vi "MGI Read Spreadsheet File.vi"(5 "Dialog pattern (*.txt)":string="*.txt", 6 "Start Offset":i64, 7 "Delimiter (Tab)":string="\t", 8 "Error In":errorcluster, 11 "Path":path) -> (0 "Error Out":errorcluster, 1 "EOF Reached?":bool, 2 "Values":dbl[][](array[numeric]) format="%_3p", 3 "Headers":string[][](array[string]), 4 "End Offset":i64)   [LabVIEW 2016]
doc: "Reads a spreadsheet file by returning the first non-empty, non numeric containing rows as a header, then the following numeric rows. Reading starts at Start Offset. End Offset is the file offset for the next Header/Values section.\nThis VI is similar to the vi.lib file \"Read From Spreadsheet File.vi\", but it supports headers.\n\nAuthored by Shawn Walpole\nsupport@mooregoodideas.com\nwww.mooregoodideas.com\n\nCopyright (c) 2010, Moore Good Ideas, Inc.\n\nAll rights reserved.\n\nRedistribution and use in source and binary forms, with or without modification, are permitted provided that the following conditions are met:\n\n * Redistributions of source code must retain the above copyright notice, this list of conditions and the following disclaimer.\n * Redistributions in binary form must reproduce the above copyright notice, this list of conditions and the following disclaimer in the documentation and/or other materials provided with the distribution.\n * Neither the name of Moore Good Ideas, Inc. nor the names of its contributors may be used to endorse or promote products derived from this software without specific prior written permission.\n\nTHIS SOFTWARE IS PROVIDED BY THE COPYRIGHT HOLDERS AND CONTRIBUTORS \"AS IS\" AND ANY EXPRESS OR IMPLIED WARRANTIES, INCLUDING, BUT NOT LIMITED TO, THE IMPLIED WARRANTIES OF MERCHANTABILITY AND FITNESS FOR A PARTICULAR PURPOSE ARE DISCLAIMED. IN NO EVENT SHALL THE COPYRIGHT OWNER OR CONTRIBUTORS BE LIABLE FOR ANY DIRECT, INDIRECT, INCIDENTAL, SPECIAL, EXEMPLARY, OR CONSEQUENTIAL DAMAGES (INCLUDING, BUT NOT LIMITED TO, PROCUREMENT OF SUBSTITUTE GOODS OR SERVICES; LOSS OF USE, DATA, OR PROFITS; OR BUSINESS INTERRUPTION) HOWEVER CAUSED AND ON ANY THEORY OF LIABILITY, WHETHER IN CONTRACT, STRICT LIABILITY, OR TORT (INCLUDING NEGLIGENCE OR OTHERWISE) ARISING IN ANY WAY OUT OF THE USE OF THIS SOFTWARE, EVEN IF ADVISED OF THE POSSIBILITY OF SUCH DAMAGE."
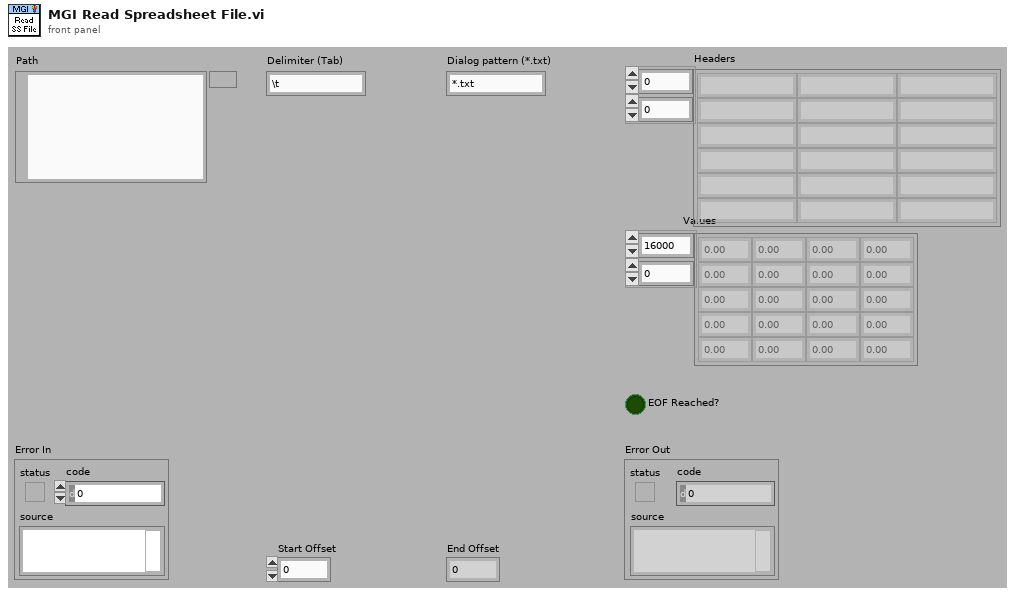
[diagram p1: front panel]
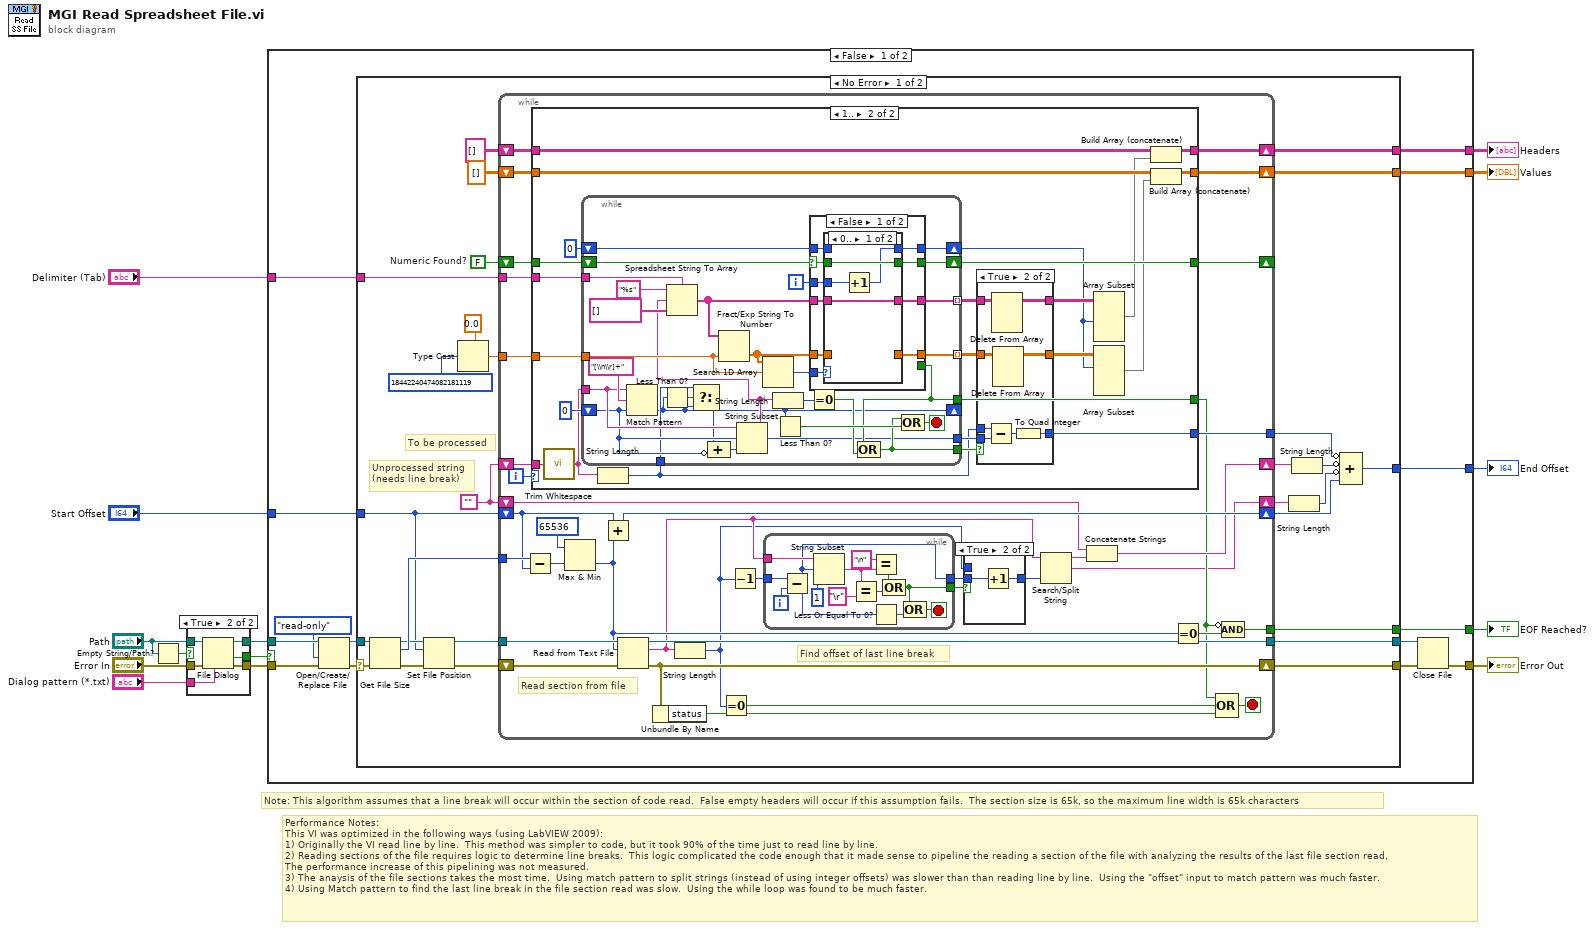
[diagram p0: block diagram]
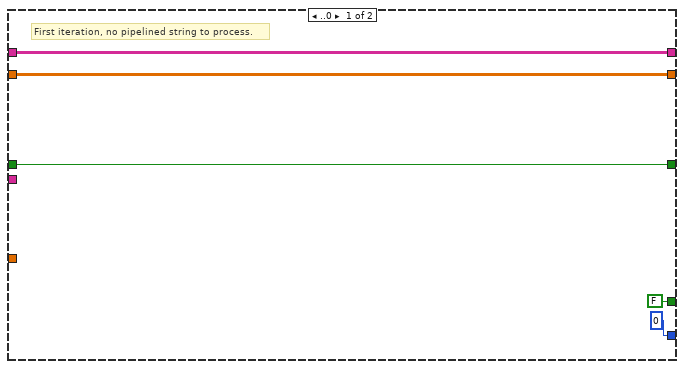
[diagram p3: hidden frame]
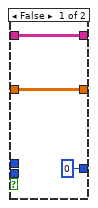
[diagram p4: hidden frame]
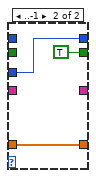
[diagram p5: hidden frame]
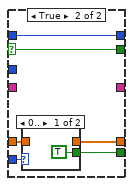
[diagram p6: hidden frame]
diagram:
  # "Note: This algorithm assumes that a line break will occur within the section of code read.  False empty headers will occur if this assumption fails.  The section size is 65k, so the maximum line width is 65k characters"
  # "Performance Notes:\nThis VI was optimized in the following ways (using LabVIEW 2009):\n1) Originally the VI read line by line.  This method was simpler to code, but it took 90% of the time just to read line by line.\n2) Reading sections of the file requires logic to determine line breaks.  This logic complicated the code enough that it made sense to pipeline the reading a section of the file with analyzing the results of the last file section read.  \nThe performance increase of this pipelining was not measured.\n3) The anaysis of the file sections takes the most time.  Using match pattern to split strings (instead of using integer offsets) was slower than than reading line by line.  Using the \"offset\" input to match pattern was much faster.\n4) Using Match pattern to find the last line break in the file section read was slow.  Using the while loop was found to be much faster."
  n1 = Empty String/Path?(string/path="Path") -> (empty?=w7:bool)
  n2 = case shown="True" w7 {
    tunnel: "Path" -> [w16 w22]
    tunnel: "Dialog pattern (*.txt)" -> [_ w21]
    tunnel: [_ w20] -> w2
    tunnel: [w15 w19] -> w4
    tunnel: "Error In" -> [w15 w18]
    tunnel: [w16 w17] -> w3
    frame False {
    }
    frame True {
      n3 = File Dialog(6:w21, 8:w18, 11:w22) -> (0:w19:errorcluster, 1:w20:bool, 3:w17:path)  [unwired: 4 in, 1 out]
    }
  }
  n4 = case shown="False" w2 {
    tunnel: [w30 _] -> w14
    tunnel: "Start Offset" -> [w28 w215]
    tunnel: [w36 _] -> w12
    tunnel: [w35 _] -> w11
    tunnel: [w29 w215] -> w10
    tunnel: [w34 _] -> w9
    tunnel: "Delimiter (Tab)" -> [w33 _]
    tunnel: w4 -> [w32 _]
    tunnel: w3 -> [w31 _]
    frame False {
      n5 = Open/Create/Replace File(file path (use dialog)=w31, error in=w32, access (0:read/write)=enum16{"read/write", "read-only", "write-only"}."read-only") -> (refnum out=w24:refnum<file>, error out=w23:errorcluster)  [unwired: 3 in, 1 out]
      n6 = case shown="No Error" w23 {
        selector: w23 -> [w62 w214]
        tunnel: [w59 w214] -> w26
        tunnel: [w39 _] -> w36
        tunnel: [w38 _] -> w35
        tunnel: [w37 _] -> w34
        tunnel: w33 -> [w41 _]
        tunnel: w24 -> [w61 w213]
        tunnel: [w53 w213] -> w25
        tunnel: [w47 w212] -> w29
        tunnel: w28 -> [w55 w212]
        frame No Error {
          w40 = FALSE  # Numeric Found?
          w52 = ""
          # "To be processed"
          # "Unprocessed string\n(needs line break)"
          n7 = Get File Size(file=w61, error in=w62) -> (refnum out=w58:refnum<file>, size (in bytes)=w60:i64, 0:w57:errorcluster)
          n8 = Set File Position(offset (in bytes) (0)=w55, refnum=w58, error in=w57) -> (refnum out=w54:refnum<file>, error out=w56:errorcluster)  [unwired: 1 in]
          n9 = Type Cast(type=0.0, x=u64 18442240474082181119) -> (*(type *) &x=w42:dbl)
          n10 = while {
            tunnel: [w74] -> w37
            tunnel: w54 -> [w101]
            tunnel: w60 -> [w99]
            shift-right: [w94] -> w59
            shift-left: w56 -> [w100]
            shift-right: [w91] -> w48
            shift-left: w55 -> [w92]
            shift-right: [w66] -> w51
            shift-left: w52 -> [w90]
            tunnel: [w93] -> w53
            shift-right: [w89] -> w50
            shift-left: w52 -> [w85]
            tunnel: [w86] -> w49
            shift-right: [w79] -> w39
            shift-left: string[][] [] -> [w84]
            shift-right: [w78] -> w38
            shift-left: dbl[][] [] -> [w83]
            tunnel: w42 -> [w82]
            tunnel: w41 -> [w81]
            shift-right: [w77] -> _
            shift-left: w40 -> [w80]
            i -> [w87]
            stop <- w95 stop-if-true
            # "Read section from file"
            # "Find offset of last line break"
            n11 = Subtract(x=w99, y=w92) -> (x-y=w98:i64)
            n12 = case shown="1.." w87 {
              tunnel: [FALSE w126] -> w73
              tunnel: [i64 0 w142] -> w86
              tunnel: w85 -> [_ w124]
              tunnel: w84 -> [w120 w141]
              tunnel: w83 -> [w119 w139]
              tunnel: w82 -> [_ w145]
              tunnel: w81 -> [_ w144]
              tunnel: w80 -> [w118 w143]
              tunnel: [w120 w140] -> w79
              tunnel: [w119 w138] -> w78
              tunnel: [w118 w136] -> w77
              frame ..0 {
                # "First iteration, no pipelined string to process."
              }
              frame 1.. {
                n13 = call <vilib>:"Trim Whitespace.vi"("string"=w124) -> ("trimmed string"=w123:string)  [unwired: 1 in]
                n14 = String Length(string=w123) -> (length=w125:i32)
                n15 = while {
                  tunnel: w145 -> [w186]
                  tunnel: w123 -> [w170]
                  shift-right: [w158] -> _
                  shift-left: 0 -> [w162]
                  tunnel: w144 -> [w180]
                  shift-right: [w174] -> w136
                  shift-left: w143 -> [w176]
                  tunnel: [w168] -> w133
                  shift-right: [w175] -> w127
                  shift-left: 0 -> [w177]
                  tunnel: [w173] -> w135 mode=indexing
                  tunnel: [w172] -> w134 mode=indexing
                  tunnel: [w162] -> w132
                  tunnel: [w164] -> w126
                  tunnel: w125 -> [w161]
                  i -> [w171]
                  stop <- w179 stop-if-true
                  n16 = Match Pattern(string=w170, regular expression="[\\n\\r]+", offset (0)=w162) -> (offset past match=w158:i32)  [unwired: 3 out]
                  n17 = Less Than 0?(x=w158) -> (x < 0?=w163:bool)
                  n18 = Select(t=w161, s=w163, f=w158) -> (s? t:f=w160:i32)
                  n19 = Compound Arithmetic op=ADD(w160, invert w162) -> (w159:i32)
                  n20 = String Subset(string=w170, offset (0)=w162, length (rest)=w159) -> (substring=w167:string)
                  n21 = Spreadsheet String To Array(delimiter (Tab)=w180, format string="%s", spreadsheet string=w167, array type (2D Dbl)=string[] []) -> (array=w181:string[])
                  n22 = Fract/Exp String To Number(string=w181, default (0 dbl)=w186) -> (number=w185:dbl[])  [unwired: 2 in, 1 out]
                  n23 = Search 1D Array(1D array=w185, element=w186) -> (index of element=w178:i32)  [unwired: 1 in]
                  n24 = String Length(string=w167) -> (length=w166:i32)
                  n25 = Less Than 0?(x=w158) -> (x < 0?=w169:bool)
                  n26 = Equal To 0?(x=w166) -> (x = 0?=w165:bool)
                  n27 = case shown="False" w176 {
                    selector: w176 -> [w192 w204]
                    tunnel: w185 -> [w189 w209]
                    tunnel: w181 -> [w195 _]
                    tunnel: w178 -> [w196 w208]
                    tunnel: w177 -> [w187 w207]
                    tunnel: w171 -> [w194 _]
                    tunnel: [w193 w207] -> w175
                    tunnel: [w191 w204] -> w174
                    tunnel: [w190 _] -> w173
                    tunnel: [w188 w205] -> w172
                    tunnel: [_ w206] -> w164
                    frame False {
                      n28 = case shown="0.." w196 {
                        tunnel: w195 -> [w199 _]
                        tunnel: w194 -> [w198 w202]
                        tunnel: [w197 w202] -> w193
                        tunnel: w192 -> [w200 _]
                        tunnel: [w200 TRUE] -> w191
                        tunnel: [w199 _] -> w190
                        tunnel: w189 -> [_ w203]
                        tunnel: [_ w203] -> w188
                        tunnel: w187 -> [_ _]
                        frame 0.. {
                          n29 = Increment(x=w198) -> (x+1=w197:i32)
                        }
                        frame ..-1 {
                        }
                      }
                    }
                    frame True {
                      n30 = case shown="0.." w208 {
                        tunnel: w209 -> [_ w211]
                        tunnel: [TRUE _] -> w206
                        tunnel: [_ w211] -> w205
                        frame 0.. {
                        }
                        frame ..-1 {
                        }
                      }
                    }
                  }
                  n31 = Compound Arithmetic op=OR(w164, w165) -> (w168:bool)
                  n32 = Compound Arithmetic op=OR(w168, w169) -> (w179:bool)
                }
                n33 = case shown="True" w133 {
                  tunnel: [i64 0 w154] -> w142
                  tunnel: w125 -> [_ w157]
                  tunnel: w135 -> [w149 w153]
                  tunnel: w134 -> [w148 w151]
                  tunnel: w132 -> [_ w156]
                  tunnel: [w149 w152] -> w130
                  tunnel: [w148 w150] -> w129
                  frame False {
                  }
                  frame True {
                    n34 = Subtract(x=w157, y=w156) -> (x-y=w155:i32)
                    n35 = Delete From Array(array=w153) -> (array with subset deleted=w152:string[][])  [unwired: 3 in, 1 out]
                    n36 = Delete From Array(array=w151) -> (array with subset deleted=w150:dbl[][])  [unwired: 3 in, 1 out]
                    n37 = To Quad Integer(1:w155) -> (0:w154:i64)
                  }
                }
                n38 = Array Subset(array=w130, length (row)=w127) -> (w131:string[][])  [unwired: 3 in]
                n39 = Array Subset(array=w129, index (row)=w127) -> (w128:dbl[][])  [unwired: 3 in]
                n40 = Build Array (concatenate)(w141, w131) -> (w140:string[][])
                n41 = Build Array (concatenate)(w139, w128) -> (w138:dbl[][])
              }
            }
            n42 = Max & Min(x=i64 65536, y=w98) -> (min(x,y)=w76:i64)  [unwired: 1 out]
            n43 = Add(x=w92, y=w76) -> (x+y=w91:i64)
            n44 = Read from Text File(file (use dialog)=w101, count=w76, error in=w100) -> (refnum out=w93:refnum<file>, text=w68:string, error out=w94:errorcluster)  [unwired: 1 in, 1 out]
            n45 = Unbundle By Name(w94) -> ("status"=w96:bool)
            n46 = String Length(string=w68) -> (length=w65:i32)
            n47 = Equal To 0?(x=w65) -> (x = 0?=w88:bool)
            n48 = Decrement(x=w65) -> (x-1=w72:i32)
            n49 = while {
              tunnel: w68 -> [w117]
              tunnel: w72 -> [w115]
              tunnel: [w108] -> w70
              tunnel: [w106] -> w69
              i -> [w114]
              stop <- w105 stop-if-true
              n50 = Subtract(x=w115, y=w114) -> (x-y=w108:i32)
              n51 = String Subset(string=w117, offset (0)=w108, length (rest)=1 ("length (rest)")) -> (substring=w112:string)
              n52 = Equal?(x=w112, y="\r" ("regular expression")) -> (x = y?=w113:bool)
              n53 = Equal?(x="\n" ("regular expression"), y=w112) -> (x = y?=w111:bool)
              n54 = Less Or Equal To 0?(x=w108) -> (x <= 0?=w107:bool)
              n55 = Compound Arithmetic op=OR(w111, w113) -> (w106:bool)
              n56 = Compound Arithmetic op=OR(w106, w107) -> (w105:bool)
            }
            n57 = case shown="True" w69 {
              tunnel: [w102 w104] -> w71
              tunnel: w70 -> [_ w103]
              tunnel: w65 -> [w102 _]
              frame False {
              }
              frame True {
                n58 = Increment(x=w103) -> (x+1=w104:i32)
              }
            }
            n59 = Search/Split String(string=w68, offset (0)=w71) -> (substring before match=w67:string, match + rest of string=w66:string)  [unwired: 1 in, 1 out]
            n60 = Concatenate Strings(w90, w67) -> (w89:string)
            n61 = Equal To 0?(x=w76) -> (x = 0?=w75:bool)
            n62 = Compound Arithmetic op=OR(w73, w88, w96) -> (w95:bool)
            n63 = Compound Arithmetic op=AND(invert w73, w75) -> (w74:bool)
          }
          n64 = String Length(string=w51) -> (length=w45:i32)
          n65 = String Length(string=w50) -> (length=w46:i32)
          n66 = Compound Arithmetic op=ADD(invert w49, invert w46, invert w45, w48) -> (w47:i64)
        }
        frame Error {
        }
      }
      n67 = Close File(refnum=w25, error in=w26) -> (error out=w30:errorcluster)  [unwired: 1 out]
    }
    frame True {
      # "Cancelled"
    }
  }
  "Values" <- w11
  "Error Out" <- w14
  "Headers" <- w12
  "End Offset" <- w10
  "EOF Reached?" <- w9
